vi "Set FPGA constants.vi"(8 "error in (no error)":errorcluster, 11 "AODAcq in":refnum<class "AODAcq.lvclass">) -> (0 "error out":errorcluster, 3 "AODAcq out":refnum<class "AODAcq.lvclass">)   [LabVIEW 2011, in "AODAcq.lvclass"]
uses:
  AODAcq.lvclass
  <vilib>/rvi/interface/RandomDataEmulation/niFpgaWriteControlTemplate.vi
  <vilib>/rvi/interface/nirviReadWriteControl/nirviReadWriteControl.xnode
  FPGA_Control/AODRef.ctl
  FPGA_Control/AOD Control (FPGA).vi
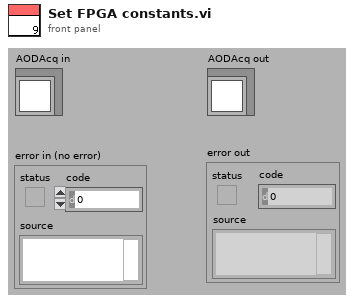
[diagram p1: front panel]
types:
  T1 = typedef "AODRef.ctl" = refnum<k20>
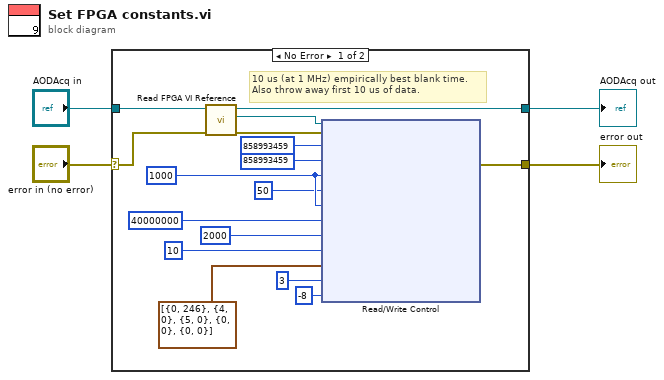
[diagram p0: block diagram]
diagram:
  n1 = case shown="No Error" "error in (no error)" {
    selector: "error in (no error)" -> [w12 w22]
    tunnel: [w11 w22] -> w3
    tunnel: [w19 w21] -> w1
    tunnel: "AODAcq in" -> [w20 w21]
    frame No Error {
      w7 = u32 1000 ("Downsample")
      # "10 us (at 1 MHz) empirically best blank time.\nAlso throw away first 10 us of data."
      n2 = call-dynamic "Read FPGA VI Reference.vi"("error in (no error)"=w12, "AODAcq in"=w20) -> ("error out"=w17:errorcluster, "FPGA VI Reference"=w18:T1, "AODAcq out"=w19:refnum<class "AODAcq.lvclass">)  [unwired: 7 in]
      n3 = xnode "Read/Write Control"("FPGA VI Reference In"=w18, "error in"=w17, "AOD.HP Center Frequency"=u32 858993459 ("LP Center Frequency"), "AOD.LP Center Frequency"=u32 858993459 ("LP Center Frequency"), "Setup.Downsample"=w7, "AOD.BlankSamples"=u16 50, "AOD.ThrowawaySamples"=w7, "Update IO timeout"=u32 40000000 ("Setup.PMT Timeout"), "AOD.UpdatesPerPoint"=u32 2000, "Comm.P high"=u32 10 ("P high"), "Debug.FinishedSetting"=cluster{"Address":u8, "Value":u32}[] [{"Address"=0, "Value"=246}, {"Address"=4, "Value"=0}, {"Address"=5, "Value"=0}, {"Address"=0, "Value"=0}, {"Address"=0, "Value"=0}], "Debug.FinishedSettingSize"=i16 3, "Setup.BitShift"=i16 -8) -> ("error out"=w11:errorcluster)  [unwired: 1 out]
    }
    frame Error {
    }
  }
  "error out" <- w3
  "AODAcq out" <- w1
